vi "parse_CMDMPC.vi"(8 "error in":errorcluster, 11 "msg in":string) -> (0 "error out":errorcluster, 2 "CMD MPC":T1, 3 "msg out":string)   [LabVIEW 2018]
uses:
  std_msgs/subs/parse_float64_scalar.vi
  <userlib>/ROS for LabVIEW Software/ROS/MessageParsing/std_msgs/subs/parse_i32_scalar.vi
  std_msgs/subs/parse_float64_array.vi
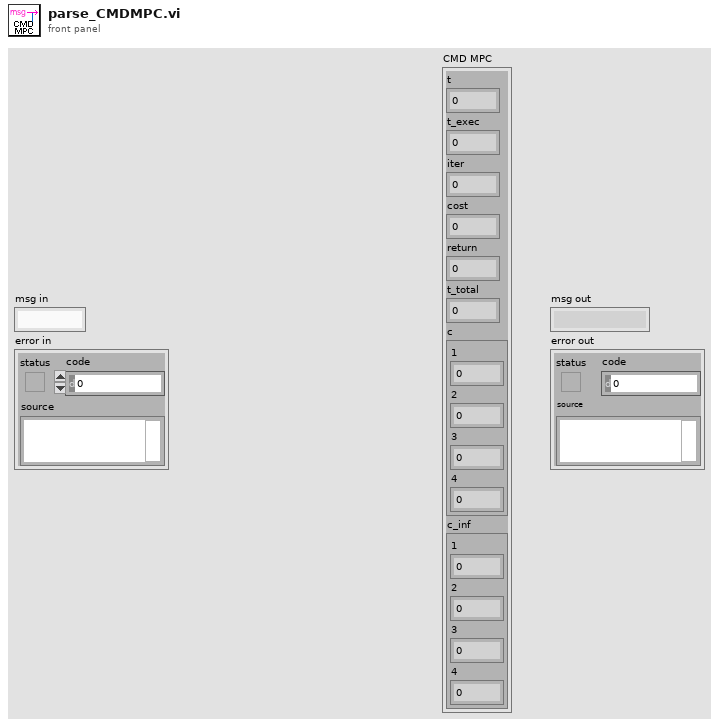
[diagram p1: front panel]
types:
  T1 = cluster{"t":dbl, "t_exec":dbl, "iter":i32, "cost":dbl, "return":i32, "t_total":dbl, "c":cluster{"1":dbl, "2":dbl, "3":dbl, "4":dbl}, "c_inf":cluster{"1":dbl, "2":dbl, "3":dbl, "4":dbl}}
  T2 = cluster{"number[0]":dbl, "number[1]":dbl, "number[2]":dbl, "number[3]":dbl}
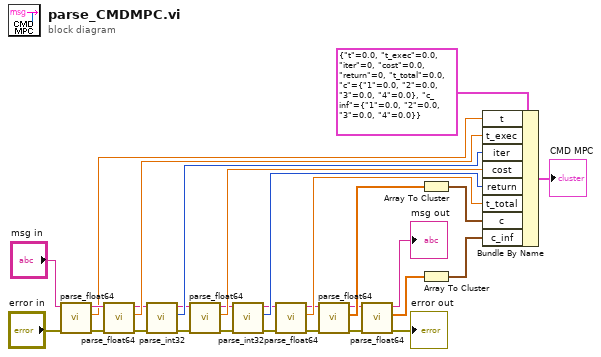
[diagram p0: block diagram]
diagram:
  n1 = call-poly "parse_float64.vi"("error in"="error in", "msg in"="msg in") -> ("error out"=w27:errorcluster, "number"=w26:dbl, "msg out"=w29:string)  [unwired: 3 in]
  n2 = call-poly "parse_float64.vi"("error in"=w27, "msg in"=w29) -> ("error out"=w21:errorcluster, "number"=w25:dbl, "msg out"=w17:string)  [unwired: 3 in]
  n3 = call-poly <userlib>:"parse_int32.vi"("error in"=w21, "msg in"=w17) -> ("error out"=w20:errorcluster, "number"=w19:i32, "msg out"=w18:string)  [unwired: 3 in]
  n4 = call-poly "parse_float64.vi"("error in"=w20, "msg in"=w18) -> ("error out"=w16:errorcluster, "number"=w24:dbl, "msg out"=w15:string)  [unwired: 3 in]
  n5 = call-poly <userlib>:"parse_int32.vi"("error in"=w16, "msg in"=w15) -> ("error out"=w13:errorcluster, "number"=w14:i32, "msg out"=w12:string)  [unwired: 3 in]
  n6 = call-poly "parse_float64.vi"("error in"=w13, "msg in"=w12) -> ("error out"=w9:errorcluster, "number"=w11:dbl, "msg out"=w10:string)  [unwired: 3 in]
  n7 = call-poly "parse_float64.vi"("error in"=w9, "msg in"=w10) -> ("error out"=w5:errorcluster, "number"=w8:dbl[], "msg out"=w6:string)  [unwired: 3 in]
  n8 = call-poly "parse_float64.vi"("error in"=w5, "msg in"=w6) -> ("error out"=→"error out":errorcluster, "number"=w2:dbl[], "msg out"=→"msg out":string)  [unwired: 3 in]
  n9 = Array To Cluster(array=w8) -> (cluster=w7:T2)
  n10 = Array To Cluster(array=w2) -> (cluster=w1:T2)
  n11 = Bundle By Name(cluster=T1 {"t"=0.0, "t_exec"=0.0, "iter"=0, "cost"=0.0, "return"=0, "t_total"=0.0, "c"={"1"=0.0, "2"=0.0, "3"=0.0, "4"=0.0}, "c_inf"={"1"=0.0, "2"=0.0, "3"=0.0, "4"=0.0}} ("MPC Info"), "t"=w26, "t_exec"=w25, "iter"=w19, "cost"=w24, "return"=w14, "t_total"=w11, "c"=w7, "c_inf"=w1) -> (→"CMD MPC":T1)
